vi "CreatePinmapWith3Pins_QueryPins_3PinsReported.vi"() -> (6 "pass":bool, 8 "result":string, 15 "error out":errorcluster)   [LabVIEW 2020]
uses:
  Pin Map Client_lv/MeasurementLink Pin Map Client/MeasurementLink Pin Map Client.lvlib
  Pin Map Client_lv/MeasurementLink Pin Map Client/RPC Messages/ni_measurementlink_pinmap_v1_CreatePinMapFromXmlRequest.ctl
  Pin Map Client_lv/MeasurementLink Pin Map Client/RPC Messages/ni_measurementlink_pinmap_v1_QueryPinsRequest.ctl
  e379b5ff-d65c-4c10-92db-bffab39ca4f8.vi
  65b5dcd1-a9b7-4222-a274-75e5d4c706a6.vi
  Pin Map Client_lv/MeasurementLink Pin Map Client/RPC Messages/ni_measurementlink_pinmap_v1_PinDefinition.ctl
panel:
  # "Test assumes discovery service and pin map service have already been started."
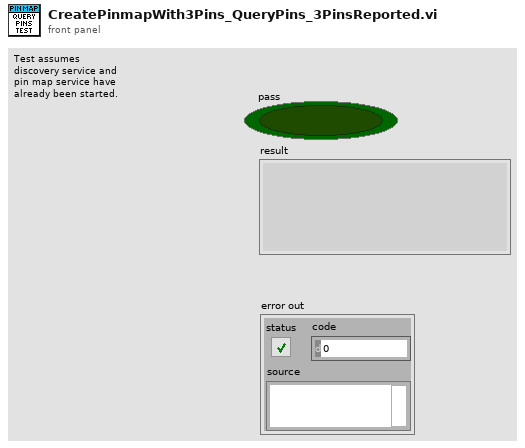
[diagram p1: front panel]
types:
  T1 = typedef "MeasurementLink Pin Map Client.lvlib/ni_measurementlink_pinmap_v1_PinDefinition.ctl" = cluster{"display_name":string, "is_system_pin":bool}
  T2 = typedef "MeasurementLink Pin Map Client.lvlib/ni_measurementlink_pinmap_v1_QueryPinsRequest.ctl" = cluster{"pin_map_id":string, "instrument_type_id":string}
  T3 = typedef "MeasurementLink Pin Map Client.lvlib/ni_measurementlink_pinmap_v1_CreatePinMapFromXmlRequest.ctl" = cluster{"pin_map_id":string, "pin_map_xml":string}
  T4 = typedef "grpc-lvsupport-release.lvlib/grpcId.ctl" = u64
  T5 = typedef "MeasurementLink Pin Map Client.lvlib/ni_measurementlink_pinmap_v1_PinMap.ctl" = cluster{"pin_map_id":string}
  T6 = typedef "MeasurementLink Pin Map Client.lvlib/ni_measurementlink_pinmap_v1_QueryPinsResponse.ctl" = cluster{"pins":T1[], "pin_groups":T7[]}
  T7 = typedef "MeasurementLink Pin Map Client.lvlib/ni_measurementlink_pinmap_v1_PinGroupDefinition.ctl" = cluster{"display_name":string, "pin_or_group_references":string[], "resolved_pins":string[]}
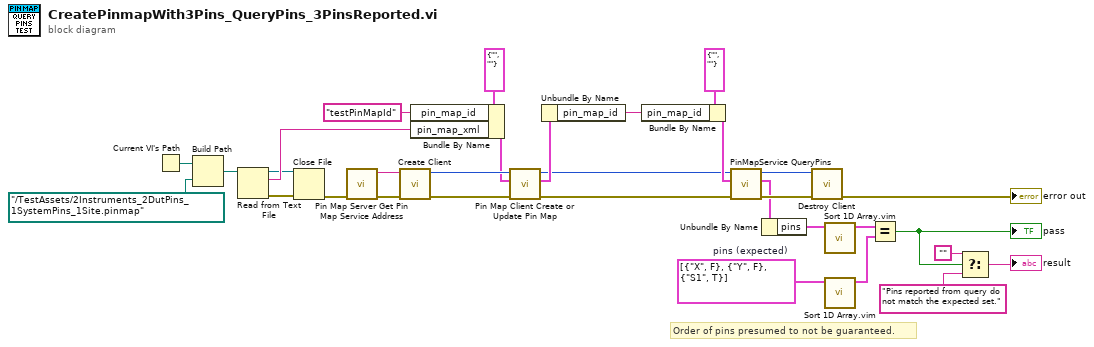
[diagram p0: block diagram]
diagram:
  w1 = T1[] [{"display_name"="X", "is_system_pin"=FALSE}, {"display_name"="Y", "is_system_pin"=FALSE}, {"display_name"="S1", "is_system_pin"=TRUE}]  # pins (expected)
  # "Order of pins presumed to not be guaranteed."
  n1 = Current VI's Path() -> (path=w30:path)
  n2 = Build Path(base path=w30, name or relative path=path "../TestAssets/2Instruments_2DutPins_1SystemPins_1Site.pinmap") -> (appended path=w28:path)
  n3 = Read from Text File(file (use dialog)=w28) -> (refnum out=w24:refnum<file>, text=w26:string, error out=w25:errorcluster)  [unwired: 3 in, 1 out]
  n4 = Close File(refnum=w24, error in=w25) -> (error out=w14:errorcluster)  [unwired: 1 out]
  n5 = call "Pin Map Server Get Pin Map Service Address.vi"("error in (no error)"=w14) -> ("error out"=w15:errorcluster, "address"=w16:string)  [unwired: 9 in]
  n6 = call "Create Client.vi"("error in"=w15, "address"=w16) -> ("error out"=w31:errorcluster, "gRPC ID Out"=w5:T4)  [unwired: 8 in]
  n7 = Bundle By Name(cluster=T3 {"pin_map_id"="", "pin_map_xml"=""} ("Request Data"), "pin_map_id"="testPinMapId", "pin_map_xml"=w26) -> (w4:T3)
  n8 = call "Pin Map Client Create or Update Pin Map.vi"("error in (no error)"=w31, "Request Data"=w4, "gRPC ID Out"=w5) -> ("error out"=w23:errorcluster, "Response Data"=w3:T5, "gRPC ID out"=w2:T4)  [unwired: 6 in]
  n9 = Unbundle By Name(w3) -> ("pin_map_id"=w19:string)
  n10 = Bundle By Name(cluster=T2 {"pin_map_id"="", "instrument_type_id"=""} ("Request Data"), "pin_map_id"=w19) -> (w18:T2)
  n11 = call "PinMapService QueryPins.vi"("error in"=w23, "Request Data"=w18, "gRPC ID"=w2) -> ("error out"=w22:errorcluster, "Response Data"=w17:T6, "gRPC ID out"=w21:T4)  [unwired: 6 in]
  n12 = Unbundle By Name(w17) -> ("pins"=w13:T1[])
  n13 = call "Destroy Client.vi"("error in"=w22, "gRPC ID"=w21) -> ("error out"=→"error out":errorcluster)  [unwired: 9 in]
  n14 = call "Sort 1D Array.vim"("unsorted array"=w13) -> ("sorted array"=w12:T1[])  [unwired: 10 in]
  n15 = call "Sort 1D Array.vim"("unsorted array"=w1) -> ("sorted array"=w11:T1[])  [unwired: 10 in]
  n16 = Equal?(x=w12, y=w11) -> (x = y?=w10:bool)
  "pass" <- w10
  n17 = Select(t="", s=w10, f="Pins reported from query do not match the expected set." ("display_name")) -> (s? t:f=→"result":string)
